vi "Open Azure Session.vi"(8 "error in (no error)":errorcluster, 11 "Credentials":T1) -> (0 "error out":errorcluster, 3 "Azure Session":refnum<class "Session.lvclass">)   [LabVIEW 2015, in "NI_Azure_Core.lvlib" / "Session.lvclass"]
doc: "Open an Azure session using the specified credentials."
uses:
  Session.lvclass
  Azure Credentials.ctl
  Session.lvclass/Session.ctl
  Write Credentials.vi
  Write HTTP Session.vi
  <vilib>/httpClient/LabVIEWHTTPClient.lvlib
  NI_Azure_Core.lvlib
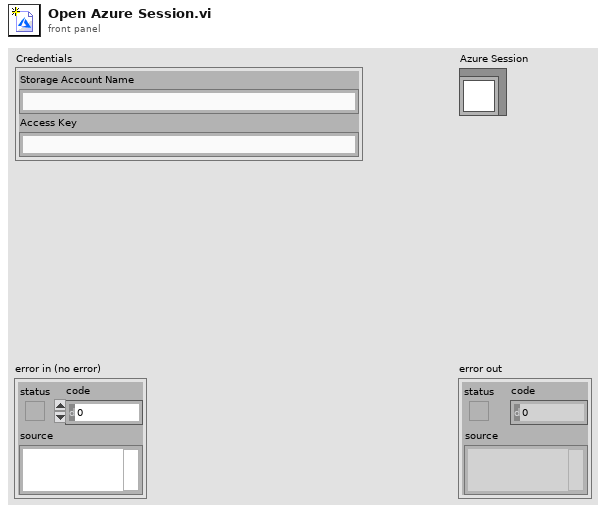
[diagram p1: front panel]
types:
  T1 = typedef "NI_Azure_Core.lvlib/Azure Credentials.ctl" = cluster{"Storage Account Name":string, "Access Key":string}
  T2 = typedef "LabVIEWHTTPClient.lvlib/ClientHandle.ctl" = refnum<k1>
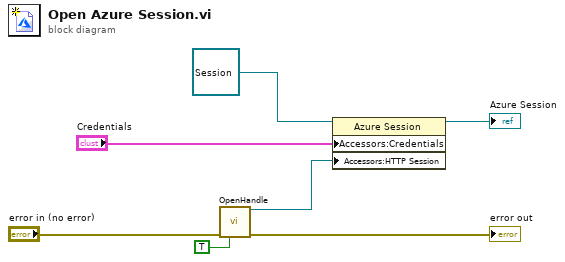
[diagram p0: block diagram]
diagram:
  n1 = call <vilib>:"OpenHandle.vi"("error in (no error)"="error in (no error)", "verify server(true)"=TRUE) -> ("client handle out"=w2:T2, "error out"=→"error out":errorcluster)  [unwired: 12 in]
  n2 = property class="Azure Session"(reference=refnum<class "Session.lvclass"> refnum ("HTTP Session"), "Accessors:Credentials"="Credentials", "Accessors:HTTP Session"=w2) -> (reference out=→"Azure Session":refnum<class "Session.lvclass">)  [unwired: 1 in, 1 out]
